vi "Delete Device from List.vi"(8 "Error In":errorcluster, 10 "Device name":string, 11 "Device List State":T1) -> (0 "Error Out":errorcluster, 3 "Device List State out":T1)   [LabVIEW 2015]
uses:
  Device List State.ctl
  Device/Device.lvclass
  Device/Read Name.vi
panel:
  out "Found":bool
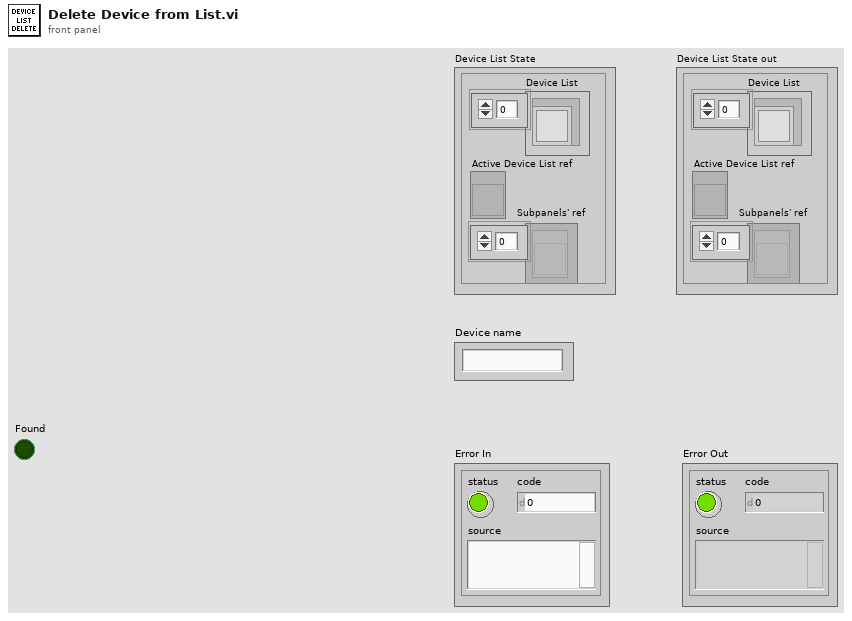
[diagram p1: front panel]
types:
  T1 = typedef "Device List State.ctl" = cluster{"Device List":refnum<class "Device.lvclass">[], "Active Device List ref":refnum<vi>, "Subpanels' ref":refnum<vi>[]}
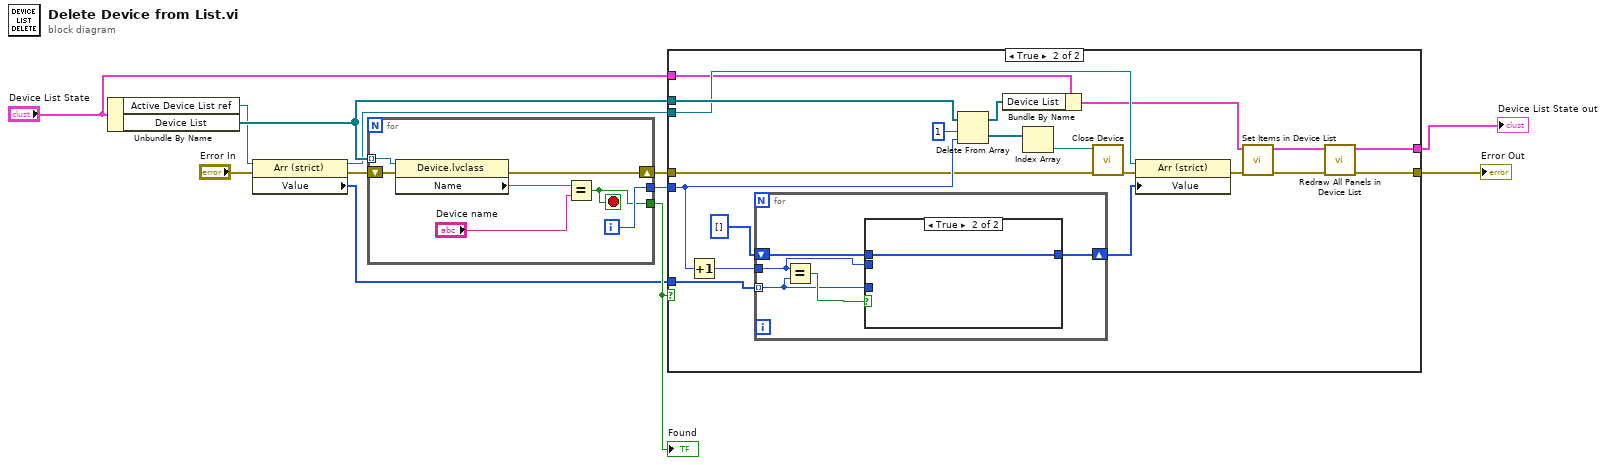
[diagram p0: block diagram]
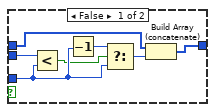
[diagram p3: hidden frame]
diagram:
  n1 = Unbundle By Name("Device List State") -> ("Active Device List ref"=w8:refnum<vi>, "Device List"=w9:refnum<class "Device.lvclass">[])
  n2 = property class="Arr (strict)"(reference=w8, error in="Error In") -> (reference out=w4:refnum<vi>, error out=w5:errorcluster, "Value"=w7:u16[])
  n3 = for {
    tunnel: w9 -> [w19] mode=indexing
    tunnel: [w17] -> w12
    tunnel: [w16] -> w11
    shift-right: [w14] -> w10
    shift-left: w5 -> [w15]
    i -> [w17]
    stop <- w16 stop-if-true
    n4 = property class="Device.lvclass"(reference=w19, error in=w15) -> (error out=w14:errorcluster, "Name"=w18:string)  [unwired: 1 out]
    n5 = Equal?(x=w18, y="Device name") -> (x = y?=w16:bool)
  }
  "Found" <- w11
  n6 = case shown="True" w11 {
    tunnel: w12 -> [_ w39]
    tunnel: w9 -> [_ w41]
    tunnel: w7 -> [_ w22]
    tunnel: w10 -> [w21 w35]
    tunnel: [w21 w26] -> w1
    tunnel: w4 -> [_ w34]
    tunnel: "Device List State" -> [w20 w32]
    tunnel: [w20 w25] -> w2
    frame False {
    }
    frame True {
      n7 = Increment(x=w39) -> (x+1=w28:i32)
      n8 = for {
        tunnel: w22 -> [w43] mode=indexing
        tunnel: w28 -> [w42]
        shift-right: [w45] -> w23
        shift-left: u16[] [] -> [w44]
        n9 = Equal?(x=w42, y=w43) -> (x = y?=w46:bool)
        n10 = case shown="True" w46 {
          tunnel: w43 -> [w49 _]
          tunnel: [w51 w54] -> w45
          tunnel: w44 -> [w50 w54]
          tunnel: w42 -> [w48 _]
          frame False {
            n11 = Less?(x=w48, y=w49) -> (x < y?=w47:bool)
            n12 = Decrement(x=w49) -> (x-1=w52:u16)
            n13 = Select(t=w52, s=w47, f=w49) -> (s? t:f=w53:u16)
            n14 = Build Array (concatenate)(w50, w53) -> (w51:u16[])
          }
          frame True {
          }
        }
      }
      n15 = Delete From Array(array=w41, length=1, index=w39) -> (deleted portion=w37:refnum<class "Device.lvclass">[], array with subset deleted=w33:refnum<class "Device.lvclass">[])
      n16 = Bundle By Name(cluster=w32, "Device List"=w33) -> (w30:T1)
      n17 = Index Array(array=w37) -> (element=w36:refnum<class "Device.lvclass">)  [unwired: 1 in]
      n18 = call "Close Device.vi"("error in (no error)"=w35, "Device"=w36) -> ("error out"=w29:errorcluster)  [unwired: 8 in, 1 out]
      n19 = property class="Arr (strict)"(reference=w34, error in=w29, "Value"=w23) -> (error out=w31:errorcluster)  [unwired: 1 out]
      n20 = call "Set Items in Device List.vi"("Error In"=w31, "Device List State"=w30) -> ("Error Out"=w27:errorcluster, "Device List State out"=w24:T1)  [unwired: 8 in]
      n21 = call "Redraw All Panels in Device List.vi"("error in (no error)"=w27, "Device List State"=w24) -> ("error out"=w26:errorcluster, "Device List State out"=w25:T1)  [unwired: 8 in]
    }
  }
  "Error Out" <- w1
  "Device List State out" <- w2
